vi "replaceControlWithItemFromNewLibrary.vi"(6 "SubVI Path":path, 8 "error in (no error)":errorcluster, 9 "Ctl Refnum":refnum<vi>, 10 "Calling VI Reference":refnum<vi>, 11 "Dependency in":refnum<class "Dependency.lvclass">) -> (0 "error out":errorcluster, 3 "Dependency out":refnum<class "Dependency.lvclass">)   [LabVIEW 2016, in "Dependency.lvclass"]
uses:
  Dependency.lvclass
  Dependency.lvclass/Dependency.ctl
  Search/Search.lvclass/Search.ctl
  Variables/CtlsReplaced.vi
  Variables/CtlsReplaceFailed.vi
  Search/Search.lvclass
  Variables/SwitchDependenciesVariables.lvlib
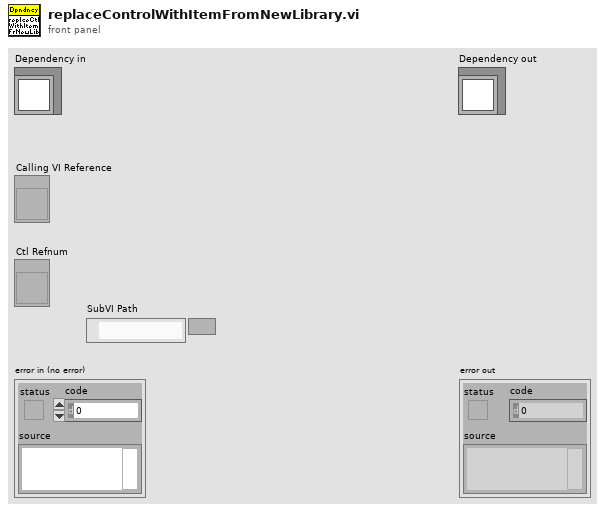
[diagram p1: front panel]
types:
  T1 = typedef "LibraryMemberNameReplacement.ctl" = cluster{"String To Replace in VI names":string, "String To Replace in Control names":string, "New String in VI names":string, "New String in Control names":string}
  T2 = typedef "LibraryDirectories.ctl" = cluster{"OldLibraryDirectory":string, "NewLibraryDirectory":string}
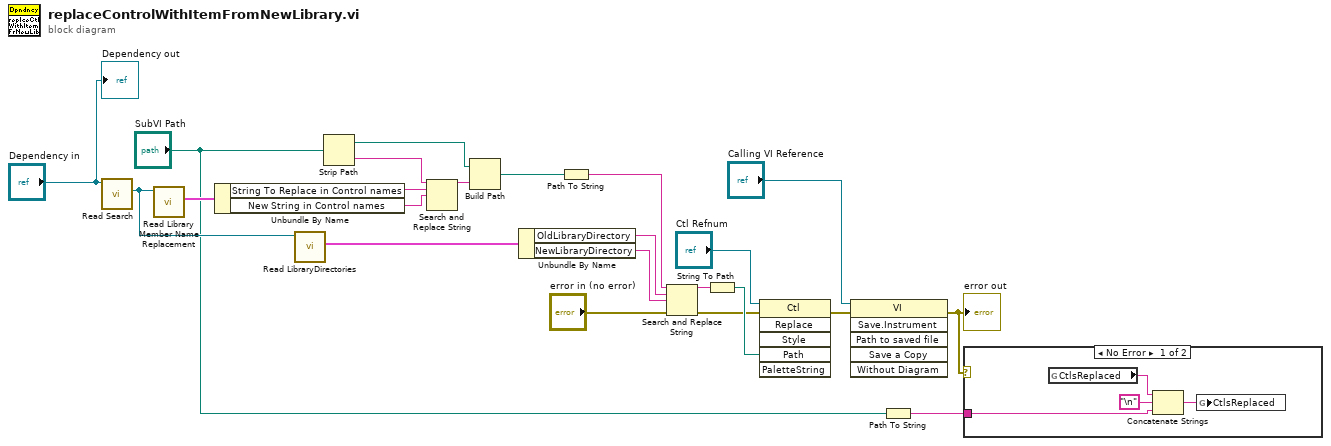
[diagram p0: block diagram]
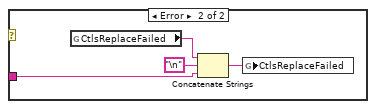
[diagram p2: hidden frame]
diagram:
  n1 = call "Read Search.vi"("Dependency in"="Dependency in") -> ("Search"=w7:refnum<class "Search.lvclass">)  [unwired: 9 in, 1 out]
  n2 = call "Read Library Member Name Replacement.vi"("ProjectItem in"=w7) -> ("Library Member Name Replacement"=w6:T1)  [unwired: 9 in, 1 out]
  n3 = Unbundle By Name(w6) -> ("String To Replace in Control names"=w19:string, "New String in Control names"=w18:string)
  n4 = call "Read LibraryDirectories.vi"("ProjectItem in"=w7) -> ("LibraryDirectories"=w8:T2)  [unwired: 9 in, 1 out]
  n5 = Strip Path(path="SubVI Path") -> (stripped path=w17:path, name=w20:string)
  n6 = Search and Replace String(input string=w20, search string=w19, replace string=w18) -> (result string=w16:string)  [unwired: 5 in, 3 out]
  n7 = Build Path(base path=w17, name or relative path=w16) -> (appended path=w15:path)
  n8 = Unbundle By Name(w8) -> ("OldLibraryDirectory"=w12:string, "NewLibraryDirectory"=w11:string)
  n9 = Path To String(path=w15) -> (string=w14:string)
  n10 = Search and Replace String(input string=w14, search string=w12, replace string=w11, error in="error in (no error)") -> (result string=w13:string, error out=w1:errorcluster)  [unwired: 4 in, 2 out]
  n11 = String To Path(string=w13) -> (path=w23:path)
  n12 = invoke class="Ctl" method="Replace"(reference="Ctl Refnum", error in=w1, "Path"=w23) -> (error out=w21:errorcluster)  [unwired: 3 in, 5 out]
  n13 = invoke class="VI" method="Save.Instrument"(reference="Calling VI Reference", error in=w21) -> (error out=w3:errorcluster)  [unwired: 4 in, 5 out]
  "error out" <- w3
  n14 = Path To String(path="SubVI Path") -> (string=w5:string)
  n15 = case shown="No Error" w3 {
    tunnel: w5 -> [w25 w29]
    frame No Error {
      n16 = global read "CtlsReplaced.vi" "CtlsReplaced"() -> (w27:string)
      n17 = Concatenate Strings(w27, "\n", w25) -> (w24:string)
      n18 = global write "CtlsReplaced.vi" "CtlsReplaced"(w24) -> ()
    }
    frame Error {
      n19 = global read "CtlsReplaceFailed.vi" "CtlsReplaceFailed"() -> (w31:string)
      n20 = Concatenate Strings(w31, "\n", w29) -> (w28:string)
      n21 = global write "CtlsReplaceFailed.vi" "CtlsReplaceFailed"(w28) -> ()
    }
  }
  "Dependency out" <- "Dependency in"
